vi "Configure Multi Eval Meas List Segment ACLR.vi"(6 "ACLR Enable (Off)":bool, 7 "ACLR Statistic Count (20)":i32=20, 8 "error in (no error)":errorcluster, 9 "Segment (1)":T1=1, 10 "Instance (1)":T2=1, 11 "VISA resource name":refnum<visa-resource-name>) -> (0 "error out":errorcluster, 3 "VISA resource name out":refnum<visa-resource-name>)   [LabVIEW 2015, in "Rohde&Schwarz CMXP NR FR2 Measurement.lvlib"]
doc: "Defines settings for ACLR measurements in list mode for segment <no>.\n\nAttribute:\nRSCMXPNRFR2M_ATTR_MULTI_EVAL_MEASUREMENT_LIST_SEGMENT_ACLR\n\nRemote-control command:\nCONFigure:NRMMw:MEAS<i>:LIST:SEGMent<no>:ACLR"
uses:
  <instrlib>/Rohde&Schwarz CMXP NR FR2 Measurement/Rohde&Schwarz CMXP NR FR2 Measurement.lvlib
  <instrlib>/Rohde&Schwarz CMXP NR FR2 Measurement/Private/_Instance.ctl
  <instrlib>/Rohde&Schwarz CMXP NR FR2 Measurement/Private/_Segment.ctl
  <instrlib>/Rohde&Schwarz CMXP NR FR2 Measurement/Private/rsidr_core.llb/rsidr_core.lvlib
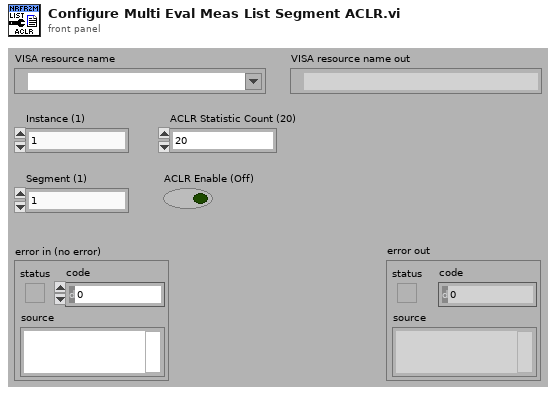
[diagram p1: front panel]
types:
  T1 = typedef "Rohde&Schwarz CMXP NR FR2 Measurement.lvlib/_Segment.ctl" = i32
  T2 = typedef "Rohde&Schwarz CMXP NR FR2 Measurement.lvlib/_Instance.ctl" = i32
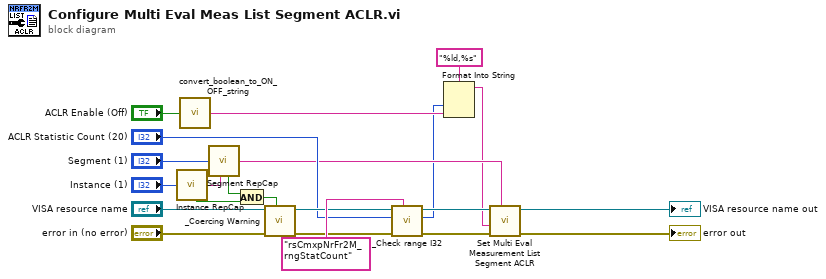
[diagram p0: block diagram]
diagram:
  n1 = call <instrlib>:"Instance RepCap.vi"("Instance In"="Instance (1)") -> ("In Range?"=w18:bool, "RepCap Identifier Out"=w3:string)  [unwired: 1 in]
  n2 = call <instrlib>:"convert_boolean_to_ON_OFF_string.vi"("boolean value in"="ACLR Enable (Off)") -> ("string value out"=w14:string)  [unwired: 4 in]
  n3 = call <instrlib>:"Segment RepCap.vi"("Segment In"="Segment (1)", "RepCap String In (\"\")"=w3) -> ("In Range?"=w17:bool, "RepCap Identifier Out"=w9:string)
  n4 = And(x=w17, y=w18) -> (x .and. y?=w19:bool)
  n5 = call <instrlib>:"_Coercing Warning.vi"("In Range?"=w19, "error in (no error)"="error in (no error)", "VISA resource name"="VISA resource name") -> ("error out"=w11:errorcluster, "VISA resource name out"=w12:refnum<visa-resource-name>)  [unwired: 7 in]
  n6 = call <instrlib>:"_Check range I32.vi"("Range Table Identifier"="rsCmxpNrFr2M_rngStatCount", "error in (no error)"=w11, "I32 Value In"="ACLR Statistic Count (20)", "VISA resource name"=w12) -> ("error out"=w7:errorcluster, "I32 Value Out"=w1:i32, "VISA resource name out"=w8:refnum<visa-resource-name>)  [unwired: 5 in]
  n7 = Format Into String(format string="%ld,%s", w1, w14) -> (resulting string=w2:string)  [unwired: 2 in, 1 out]
  n8 = call "Set Multi Eval Measurement List Segment ACLR"("Repeated Capabilities"=w9, "error in (no error)"=w7, "Multi Eval Measurement List Segment ACLR ()"=w2, "instrument handle"=w8) -> ("error out"=→"error out":errorcluster, "instrument handle out"=→"VISA resource name out":refnum<visa-resource-name>)  [unwired: 6 in]
